vi "Read Destinations.vi"(8 "error in (no error)":errorcluster, 11 "SignalManager in":refnum<class "SignalManager.lvclass">) -> (0 "error out":errorcluster, 2 "Destinations":string[](array[string]), 3 "SignalManager out":refnum<class "SignalManager.lvclass">)   [LabVIEW 2020, in "SignalManager.lvclass"]
uses:
  SignalManager.lvclass
  SignalManager.lvclass/SignalManager.ctl
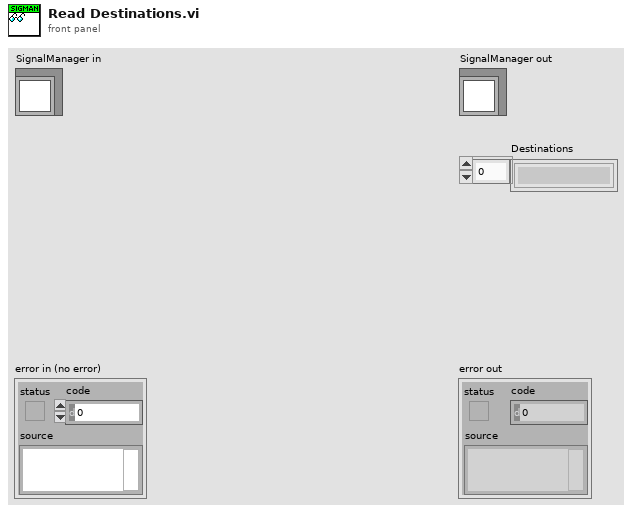
[diagram p1: front panel]
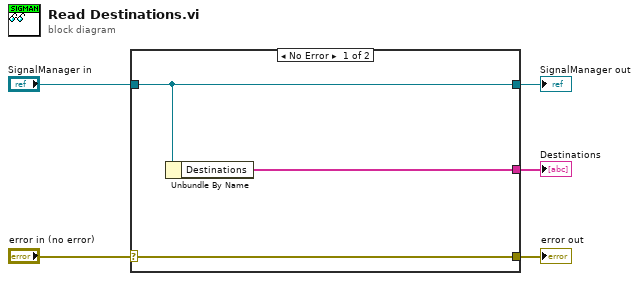
[diagram p0: block diagram]
diagram:
  n1 = case shown="No Error" "error in (no error)" {
    selector: "error in (no error)" -> [w8 w9]
    tunnel: [w8 w9] -> w4
    tunnel: [w7 w10] -> w2
    tunnel: "SignalManager in" -> [w7 w10]
    tunnel: [w6 _] -> w1
    frame No Error {
      n2 = Unbundle By Name(w7) -> ("Destinations"=w6:string[])
    }
    frame Error {
    }
  }
  "error out" <- w4
  "SignalManager out" <- w2
  "Destinations" <- w1
